vi "Send VHMI-recieveConnectionInfo.vi"(7 "Message Priority (Normal)":T2=enum."Normal", 8 "error in (no error)":errorcluster, 10 "connection status":T1, 11 "Message Enqueuer":refnum<class "Message Enqueuer.lvclass">) -> (0 "error out":errorcluster, 3 "Message Enqueuer out":refnum<class "Message Enqueuer.lvclass">)   [LabVIEW 2020, in "VHMI-VNA_Hardware_manager_Interface.lvlib" / "VHMI-recieveConnectionInfo Msg.lvclass"]
doc: "This VI sends the message to an actor."
uses:
  VHMI-recieveConnectionInfo Msg.lvclass
  <vilib>/ActorFramework/Message Enqueuer/Message Enqueuer.lvclass
  C:/Program Files (x86)/National Instruments/LabVIEW 2020/vi.lib/ActorFramework/Message/Message.lvclass
  C:/projects/VNA/src/LabVIEW/actor/hardware_manager/VHMI-VNA_Hardware_manager_Interface Messages/VHMI-recieveConnectionInfo Msg/VHMI-recieveConnectionInfo Msg.lvclass
  <vilib>/ActorFramework/Message Enqueuer/Message Priority.ctl
  VHM-VNA_Hardware_Manager/VHM-VNA_Hardware_Manager/VHM-connection_status.ctl
  VHM-VNA_Hardware_Manager/VHM-VNA_Hardware_Manager/VHM-VNA_Hardware_Manager.lvclass
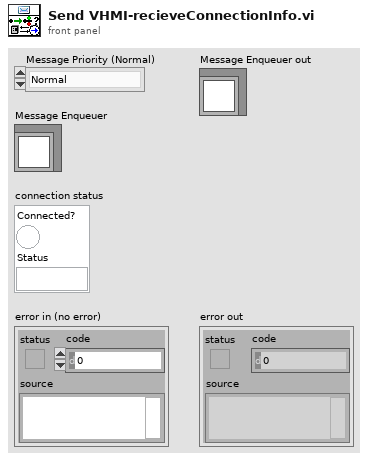
[diagram p1: front panel]
types:
  T1 = typedef "VHM-VNA_Hardware_Manager.lvlib/VHM-VNA_Hardware_Manager.lvclass/VHM-connection_status.ctl" = cluster{"Connected?":bool, "Status":string}
  T2 = typedef "Actor Framework.lvlib/Message Enqueuer.lvclass/Message Priority.ctl" = enum16{"Low", "Normal", "High"}
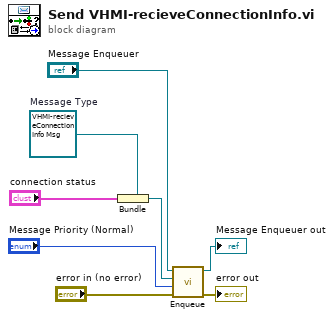
[diagram p0: block diagram]
diagram:
  w5 = refnum<class "VHMI-recieveConnectionInfo Msg.lvclass"> refnum  # Message Type
  n1 = Bundle(cluster=w5, "connection status") -> (w4:refnum<class "VHMI-recieveConnectionInfo Msg.lvclass">)
  n2 = call <vilib>:"Enqueue.vi"("error in (no error)"="error in (no error)", "Message Priority (Normal)"="Message Priority (Normal)", "Message"=w4, "Message Enqueuer in"="Message Enqueuer") -> ("error out"=→"error out":errorcluster, "Message Enqueuer out"=→"Message Enqueuer out":refnum<class "Message Enqueuer.lvclass">)  [unwired: 6 in]
